vi "Find Target Actor.vi"(5 "Target":refnum<vi>, 7 "App Inst":refnum<vi>, 8 "error in (no error)":errorcluster, 11 "Message Path":path) -> (0 "error out":errorcluster, 3 "Targeted Actor":path)   [LabVIEW 2020, in "Message Rescripter.lvlib"]
uses:
  Message Rescripter.lvlib
  <vilib>/ErrorRing/Error Ring.xnode
  <vilib>/Utility/traverseref.llb/TRef TravTarget.ctl
  <vilib>/Utility/traverseref.llb/VI Scripting - Traverse.lvlib
  <vilib>/Utility/Data Type/NI_Data Type.lvlib
  MessageMakerProvider/AFPP Shared/AFPP Shared.lvlib
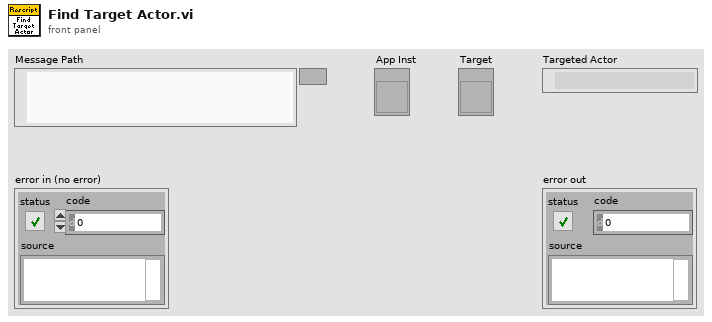
[diagram p1: front panel]
types:
  T1 = typedef "TRef TravTarget.ctl" = enum16{"FP", "BD", "Other"}
  T2 = typedef "NI_FileType.lvlib/LVFileType.ctl" = enum32{"Invalid file", "Unknown type", "Instrument", "Control", "Polymorphic VI", "Project", "Library", "LVClass", "XControl", "XNode", "Shared library", ".NET assembly", "ActiveX interface", "CIN", "Run-time menu", "Palette menu", "Help file", "LLB", "XNode Edit Dependency", "Class Private Data Control", "Statechart", "MathScript .m file", "Ladder Diagram", "LVLibp", "XNode Build Dependency"}
  T3 = cluster{"path":path, "delimited name":string, "type":T2}[]
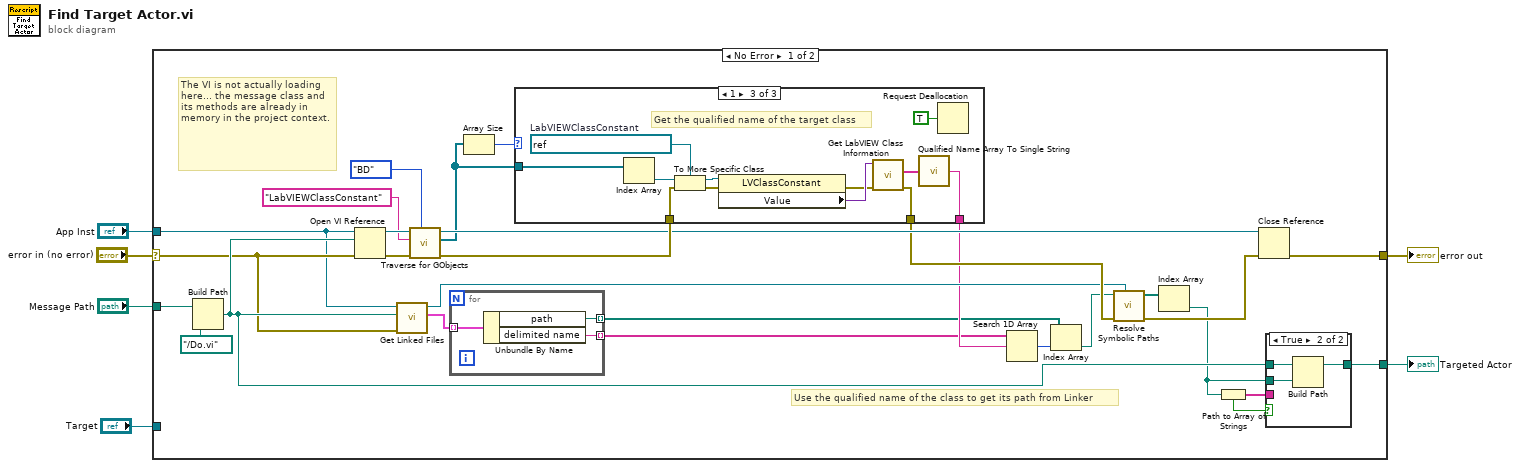
[diagram p0: block diagram]
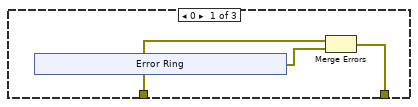
[diagram p2: hidden frame]
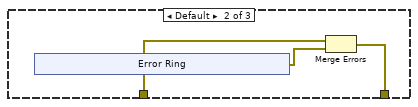
[diagram p3: hidden frame]
diagram:
  n1 = case shown="No Error" "error in (no error)" {
    selector: "error in (no error)" -> [w31 w62]
    tunnel: "Message Path" -> [w34 _]
    tunnel: [w11 _] -> w5
    tunnel: "App Inst" -> [w15 _]
    tunnel: [w30 w62] -> w3
    tunnel: "Target" -> [_ _]
    frame No Error {
      # "Use the qualified name of the class to get its path from Linker"
      # "The VI is not actually loading here... the message class and its methods are already in memory in the project context."
      n2 = Build Path(base path=w34, name or relative path=path "../Do.vi") -> (appended path=w32:path)
      n3 = Open VI Reference(application reference (local)=w15, vi path=w32, error in (no error)=w31) -> (vi reference=w29:refnum<vi>, error out=w28:errorcluster)  [unwired: 3 in]
      n4 = call "Get Linked Files.vi"("error in (no error)"=w31, "File path"=w32, "Application in"=w15) -> ("Linked Files"=w10:T3, "Application out"=w21:refnum<vi>)  [unwired: 7 in]
      n5 = call <vilib>:"Traverse for GObjects.vi"("Traverse Target"=TRef_TravTarget."BD", "error in (no error)"=w28, "Class Name"="LabVIEWClassConstant", "VI Refnum"=w29) -> ("error out"=w25:errorcluster, "References"=w14:refnum<vi>[], "dup VI Refnum"=w24:refnum<vi>)  [unwired: 4 in, 1 out]
      n6 = for {
        tunnel: w10 -> [w37] mode=indexing
        tunnel: [w36] -> w9 mode=indexing
        tunnel: [w35] -> w8 mode=indexing
        n7 = Unbundle By Name(w37) -> ("path"=w35:path, "delimited name"=w36:string)
      }
      n8 = Array Size(array=w14) -> (size(s)=w13:i32)
      n9 = case shown="1" w13 {
        tunnel: w25 -> [w40 w44 w55]
        tunnel: [w39 w43 w50] -> w22
        tunnel: [_ _ w48] -> w12
        tunnel: w14 -> [_ _ w46]
        frame 0 {
          n10 = xnode "Error Ring"() -> ("error out"=w38:errorcluster)
          n11 = Merge Errors(w40, w38) -> (w39:errorcluster)
        }
        frame Default {
          n12 = xnode "Error Ring"() -> ("error out"=w42:errorcluster)
          n13 = Merge Errors(w44, w42) -> (w43:errorcluster)
        }
        frame 1 {
          w57 = refnum<vi> refnum  # LabVIEWClassConstant
          # "Get the qualified name of the target class"
          n14 = Index Array(array=w46) -> (element=w53:refnum<vi>)  [unwired: 1 in]
          n15 = To More Specific Class(target class=w57, reference=w53, error in=w55) -> (specific class reference=w56:refnum<vi>, error out=w54:errorcluster)
          n16 = property class="LVClassConstant"(reference=w56, error in=w54) -> (error out=w51:errorcluster, "Value"=w52:variant)  [unwired: 1 out]
          n17 = call <vilib>:"Get LabVIEW Class Information.vi"("error in (no error)"=w51, "variant"=w52) -> ("error out"=w50:errorcluster, "qualified LabVIEW class name"=w49:string[])  [unwired: 7 in, 1 out]
          n18 = call <vilib>:"Qualified Name Array To Single String.vi"("Fully Qualified Array"=w49) -> ("Fully Qualified String"=w48:string)
          n19 = Request Deallocation(TRUE ("flag")) -> ()
        }
      }
      n20 = Search 1D Array(1D array=w9, element=w12) -> (index of element=w23:i32)  [unwired: 1 in]
      n21 = Index Array(array=w8, index=w23) -> (element=w20:path)
      n22 = call "Resolve Symbolic Paths.vi"("App Inst"=w21, "error in (no error)"=w22, "Path"=w20) -> ("error out"=w19:errorcluster, "Resolved Paths"=w16:path[])  [unwired: 7 in]
      n23 = Index Array(array=w16) -> (element=w7:path)  [unwired: 1 in]
      n24 = Path to Array of Strings(0:w7) -> (1:w17:bool, 2:w18:string[])
      n25 = Close Reference(reference=w24, error in (no error)=w19) -> (error out=w30:errorcluster)
      n26 = case shown="True" w17 {
        tunnel: w7 -> [w58 w59]
        tunnel: w18 -> [_ _]
        tunnel: w32 -> [_ w61]
        tunnel: [w58 w60] -> w11
        frame False {
        }
        frame True {
          n27 = Build Path(base path=w61, name or relative path=w59) -> (appended path=w60:path)
        }
      }
    }
    frame Error {
    }
  }
  "Targeted Actor" <- w5
  "error out" <- w3
